vi "Backlash.vi"   [LabVIEW 2017, in "NI_AdvCtrl_nonlinear.lvlib"]
doc: "LabVIEW no longer supports this VI. You can obtain similar functionality by installing the LabVIEW Simulation Module.\n\nImplements a backlash or deadband function. Output will not change until the input value differs from the current output by at least the deadband amount."
uses:
  <vilib>/addons/control/advanced/NI_AdvCtrl_nonlinear.lvlib
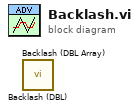
[diagram p0: block diagram]
diagram:
  n1 = call <vilib>:"Backlash (DBL).vi"() -> ()  [unwired: 4 in, 1 out]
  n2 = call <vilib>:"Backlash (DBL Array).vi"() -> ()  [unwired: 4 in, 1 out]
